vi "Ball Vision Align.vi"(10 "Dashboard Drivetrain Command":T3 {"Vision PID gains"."derivative time (Td, min)" format="%.3f"; "Vision PID gains"."integral time (Ti, min)" format="%.3f"; "Vision PID gains"."proportional gain (Kc)" format="%.3f"}, 11 "Ball Vision Packet":T1) -> ()   [LabVIEW 2015]
uses:
  <vilib>/addons/control/pid/NI_PID_pid.lvlib
  <vilib>/addons/control/pid/pid.llb/PID (DBL).vi
  Common Code/Drivetrain Vision.ctl
  Common Code/Dashboard Drivetrain Command.ctl
  Common Code/Tracking Mode.ctl
  Common Code/Ball Vision Packet.ctl
panel:
  out "Aligned?":bool
  out "X out":dbl
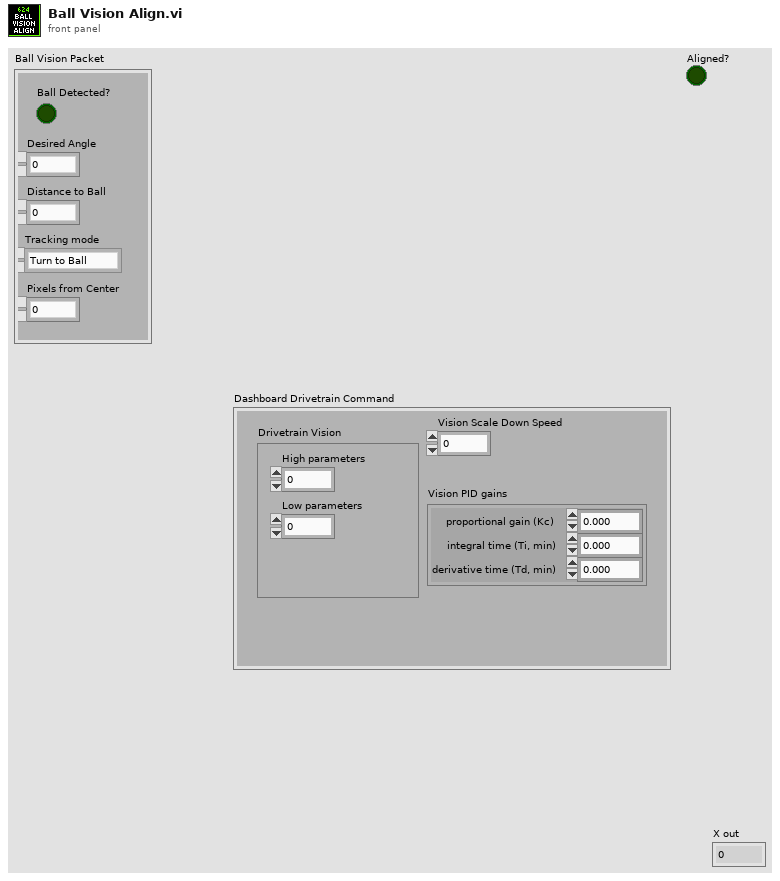
[diagram p1: front panel]
types:
  T1 = typedef "Ball Vision Packet.ctl" = cluster{"Ball Detected?":bool, "Distance to Ball":dbl, "Desired Angle":dbl, "Pixels from Center":dbl, "Tracking mode":T2}
  T2 = typedef "Tracking Mode.ctl" = enum16{"Turn to Ball", "Turn to Angle"}
  T3 = typedef "Dashboard Drivetrain Command.ctl" = cluster{"Drivetrain Vision":T4, "Vision Scale Down Speed":dbl, "Vision PID gains":cluster{"proportional gain (Kc)":dbl, "integral time (Ti, min)":dbl, "derivative time (Td, min)":dbl}}
  T4 = typedef "Drivetrain Vision.ctl" = cluster{"High parameters":dbl, "Low parameters":dbl}
  T5 = cluster{"proportional gain (Kc)":dbl, "integral time (Ti, min)":dbl, "derivative time (Td, min)":dbl}
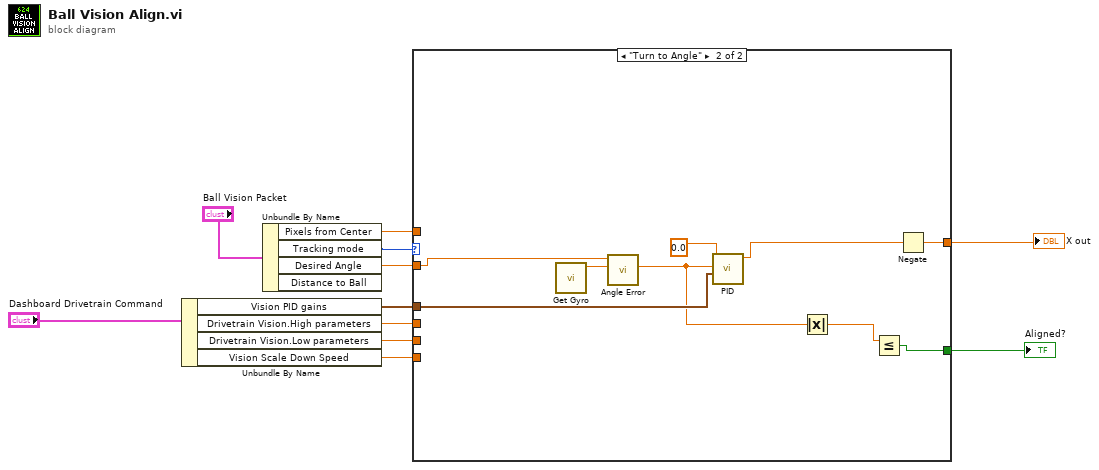
[diagram p0: block diagram]
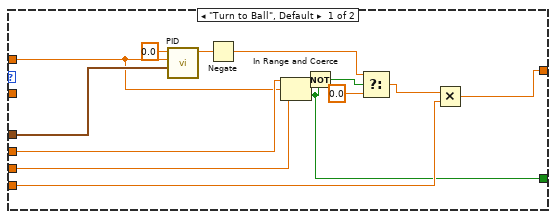
[diagram p2: hidden frame]
diagram:
  n1 = Unbundle By Name("Dashboard Drivetrain Command") -> ("Vision PID gains"=w7:T5, "Drivetrain Vision.High parameters"=w6:dbl, "Drivetrain Vision.Low parameters"=w5:dbl, "Vision Scale Down Speed"=w2:dbl)
  n2 = Unbundle By Name("Ball Vision Packet") -> ("Pixels from Center"=w3:dbl, "Tracking mode"=w9:T2, "Desired Angle"=w8:dbl)  [unwired: 1 out]
  n3 = case shown="\"Turn to Angle\"" w9 {
    tunnel: w8 -> [_ w33]
    tunnel: w7 -> [w23 w30]
    tunnel: w6 -> [w16 _]
    tunnel: w5 -> [w15 _]
    tunnel: [w19 w29] -> w4
    tunnel: w3 -> [w14 _]
    tunnel: w2 -> [w18 _]
    tunnel: [w12 w26] -> w1
    frame "Turn to Ball", Default {
      n4 = call-poly <vilib>:"PID.vi"("PID gains"=w23, "process variable"=w14, "setpoint"=0.0) -> ("output"=w22:dbl)  [unwired: 7 in, 1 out]
      n5 = Negate(x=w22) -> (-x=w21:dbl)
      n6 = In Range and Coerce(upper limit=w16, x=w14, lower limit=w15) -> (In Range?=w12:bool)  [unwired: 1 out]
      n7 = Not(x=w12) -> (.not. x?=w13:bool)
      n8 = Select(t=w21, s=w13, f=0.0) -> (s? t:f=w20:dbl)
      n9 = Multiply(x=w20, y=w18) -> (x*y=w19:dbl)
    }
    frame "Turn to Angle" {
      n10 = call "Get Gyro.vi"() -> ("Angle"=w32:dbl)  [unwired: 11 in]
      n11 = call "Angle Error.vi"("Angle"=w32, "Target Angle"=w33) -> ("Error"=w27:dbl)  [unwired: 9 in]
      n12 = call-poly <vilib>:"PID.vi"("PID gains"=w30, "process variable"=w27, "setpoint"=0.0) -> ("output"=w28:dbl)  [unwired: 7 in, 1 out]
      n13 = Absolute Value(x=w27) -> (abs(x)=w25:dbl)
      n14 = Less Or Equal?(x=w25) -> (x <= y?=w26:bool)  [unwired: 1 in]
      n15 = Negate(x=w28) -> (-x=w29:dbl)
    }
  }
  "X out" <- w4
  "Aligned?" <- w1
